vi "Main.vi"() -> ()   [LabVIEW 2020]
doc: "Use this template to build a simple state machine design pattern. Each state executes code and determines which state to transition to."
uses:
  controls/String Selector Control.ctl
  controls/State.ctl
  <vilib>/express/express analysis/Spectral/Block/exnSpectralBlock spectral measurements peak poly.vi
  <vilib>/express/express analysis/Spectral/Block/exnSpectralBlock spectral measurements peak DDT.vi
  <vilib>/express/express analysis/Spectral/XNode/ExpressSpectralMeasurementsBlockNode.xnode
panel:
  in  "Chord Detector":bool
  in  "Single String Tuning":bool
  in  "Mode Switch":bool
  out "Frequency Spectrum":dynamicdata(graph)
  in  "String Selector":T1
  out "Chord":T2
  out "Note":T3
  out "Tuner":T4
  in  "Exit":bool
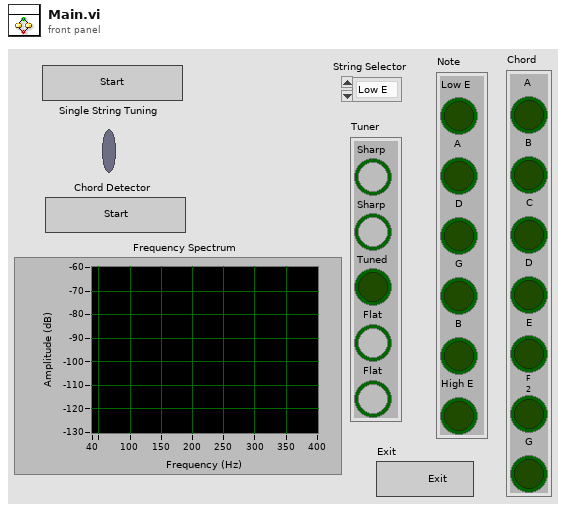
[diagram p1: front panel]
types:
  T1 = typedef "String Selector Control.ctl" = enum16{"Low E", "A", "D", "G", "B", "High E"}
  T2 = cluster{"A":bool, "B":bool, "C":bool, "D":bool, "E":bool, "F 2":bool, "G":bool}
  T3 = cluster{"Low E":bool, "A":bool, "D":bool, "G":bool, "B":bool, "High E":bool}
  T4 = cluster{"Sharp":bool, "Sharp":bool, "Tuned":bool, "Flat":bool, "Flat":bool}
  T5 = cluster{"Tuner":cluster{"Sharp":bool, "Sharp":bool, "Tuned":bool, "Flat":bool, "Flat":bool}, "Chord":cluster{"A":bool, "B":bool, "C":bool, "D":bool, "E":bool, "F 2":bool, "G":bool}, "Note":cluster{"Low E":bool, "A":bool, "D":bool, "G":bool, "B":bool, "High E":bool}, "Frequency Spectrum 2":dynamicdata}
  T6 = typedef "State.ctl" = enum16{"Initialize", "Wait for Event", "Data Acquisition", "Single String", "Chord", "Exit"}
  T7 = cluster{"averaging mode":u16, "weighting mode":u16, "number of averages":u32}
  T8 = cluster{"dB On (F)":bool, "unwrap phase (F)":bool, "convert to degree (F)":bool}
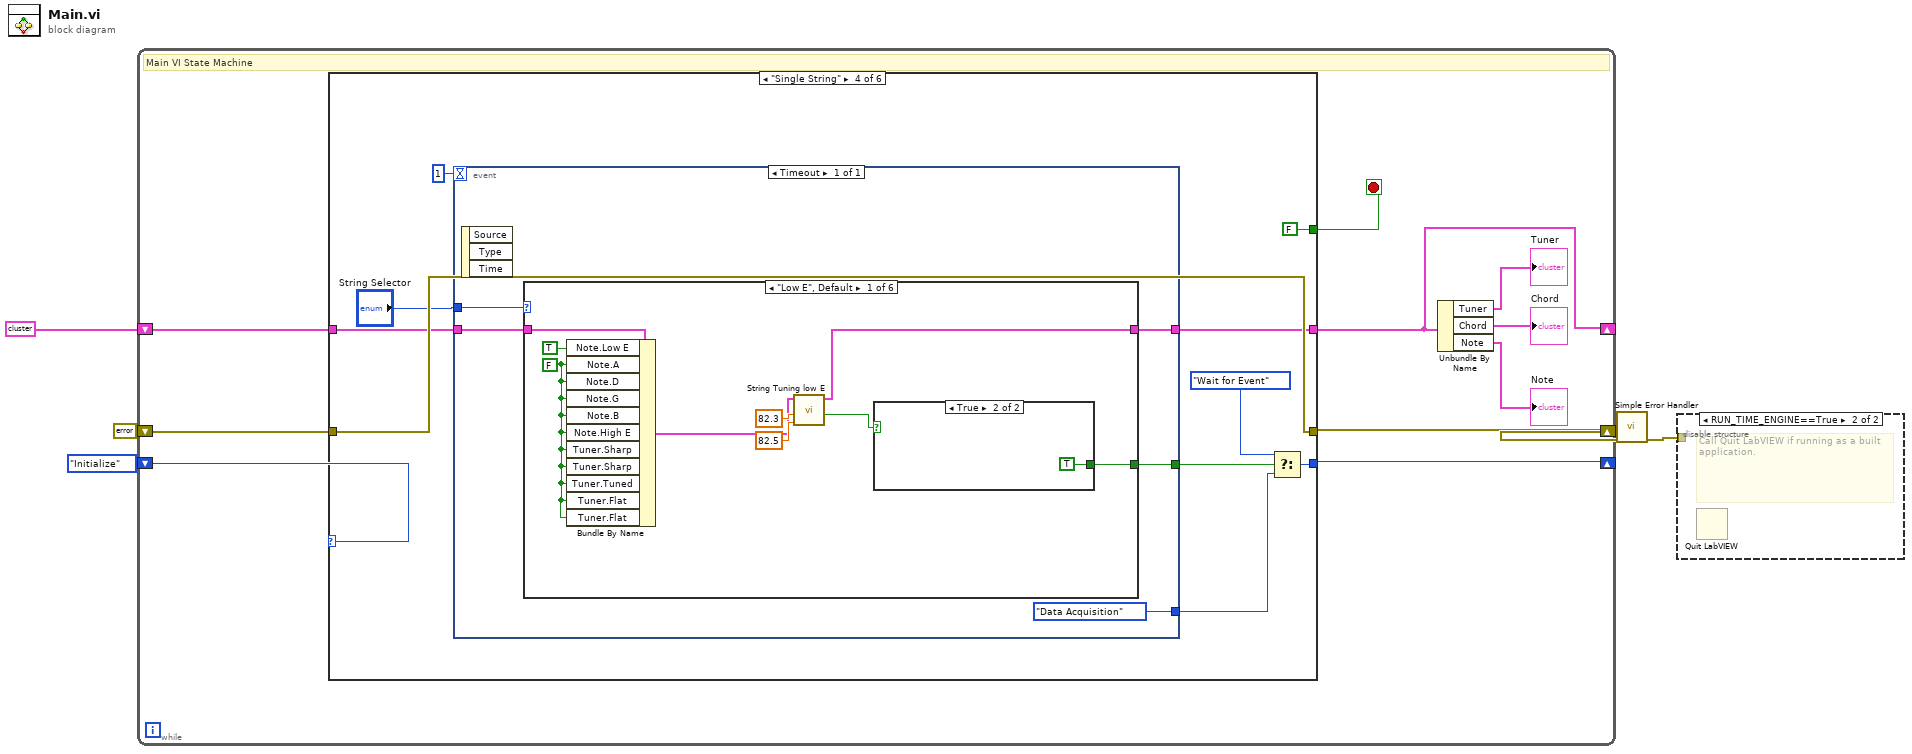
[diagram p0: block diagram]
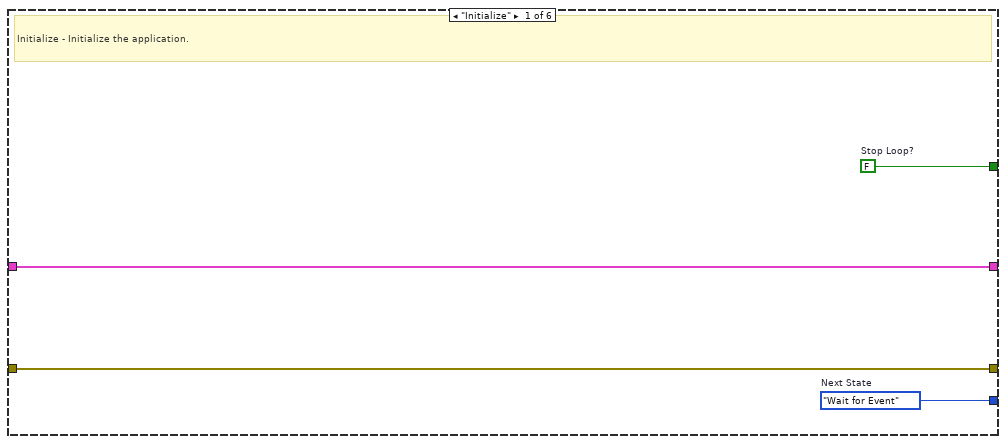
[diagram p3: hidden frame]
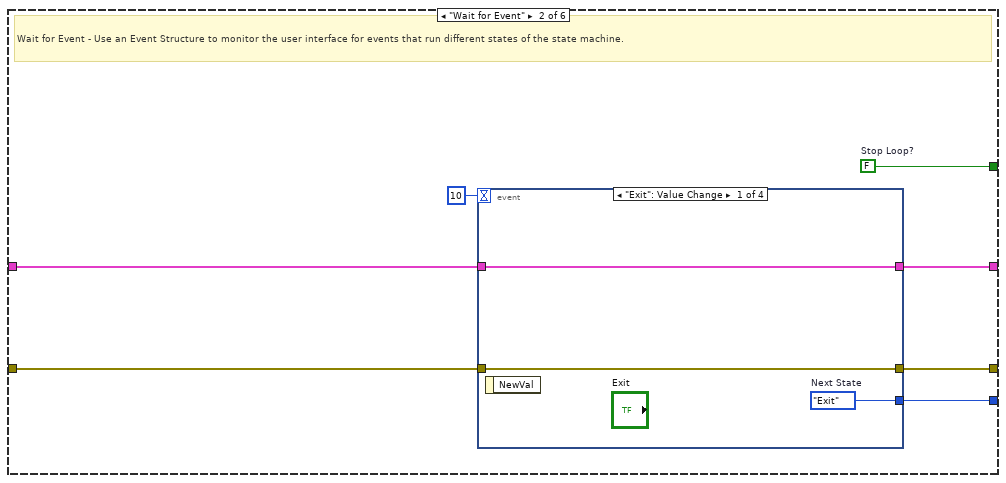
[diagram p4: hidden frame]
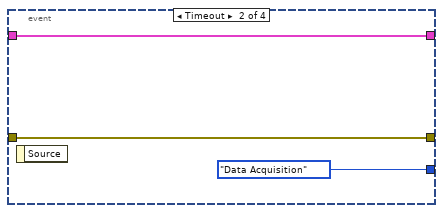
[diagram p5: hidden frame]
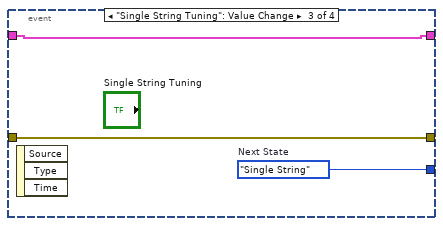
[diagram p6: hidden frame]
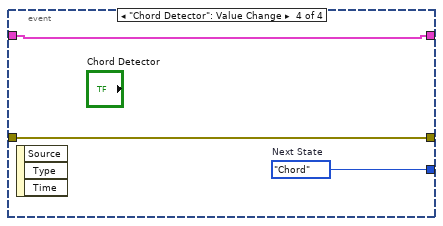
[diagram p7: hidden frame]
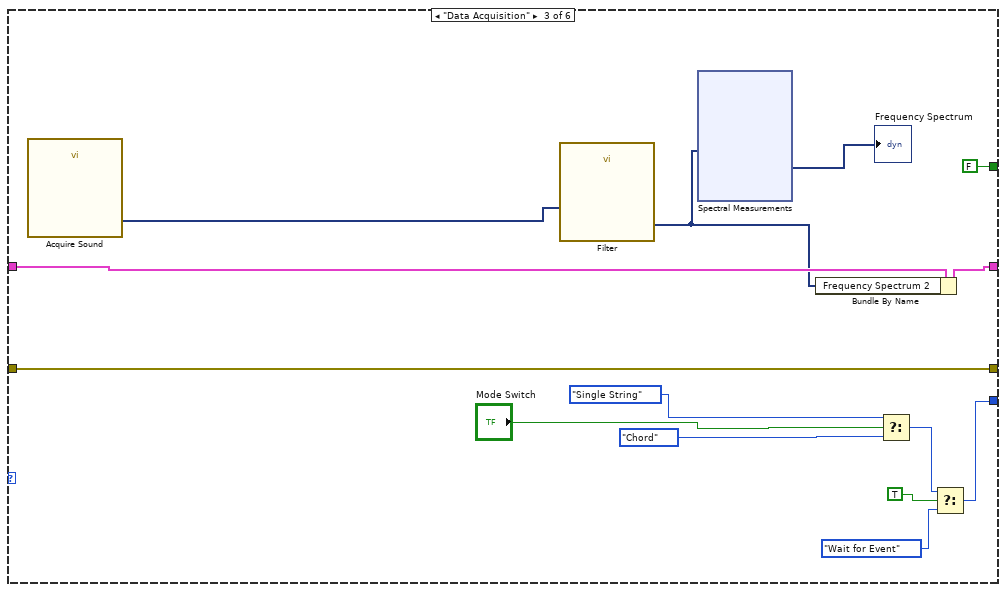
[diagram p8: hidden frame]
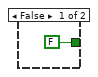
[diagram p9: hidden frame]
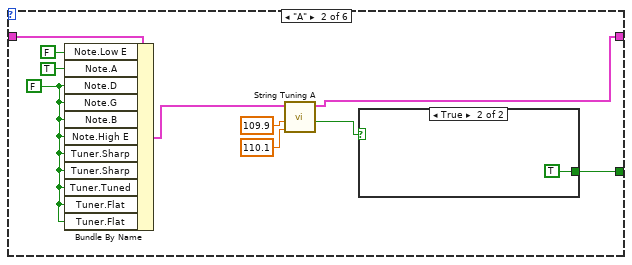
[diagram p10: hidden frame]
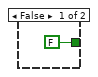
[diagram p11: hidden frame]
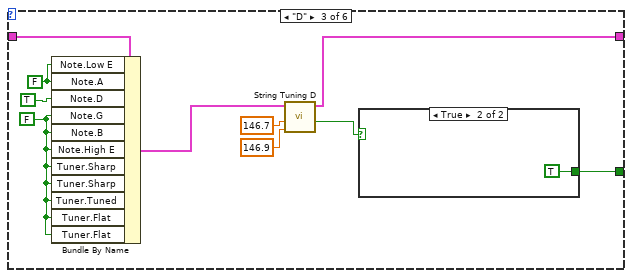
[diagram p12: hidden frame]
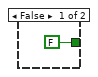
[diagram p13: hidden frame]
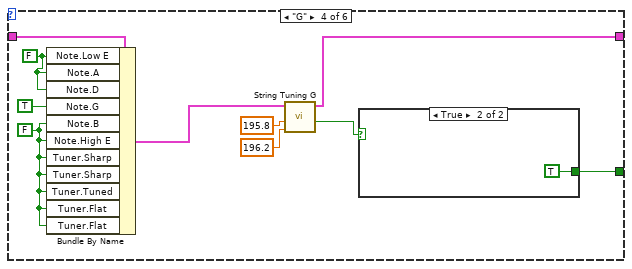
[diagram p14: hidden frame]
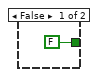
[diagram p15: hidden frame]
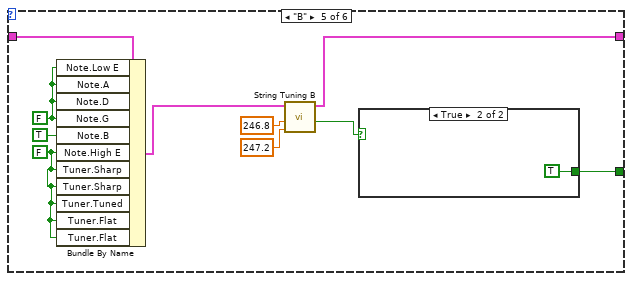
[diagram p16: hidden frame]
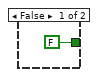
[diagram p17: hidden frame]
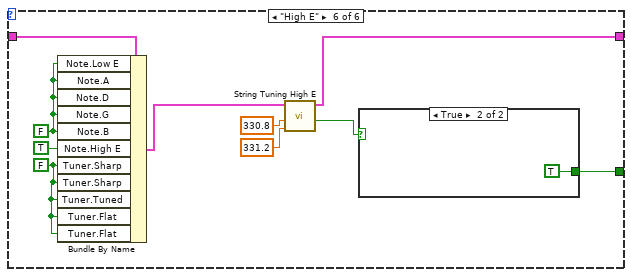
[diagram p18: hidden frame]
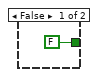
[diagram p19: hidden frame]
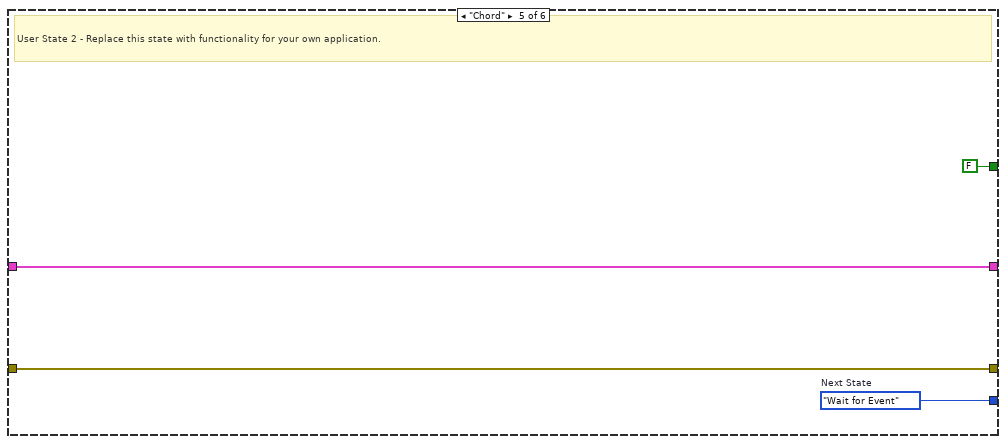
[diagram p20: hidden frame]
diagram:
  n1 = while {
    shift-right: [w14] -> _
    shift-left: State."Initialize" ("Initial State") -> [w15]
    shift-right: [w10] -> _
    shift-left: T5 {"Tuner"={"Sharp"=FALSE, "Sharp"=FALSE, "Tuned"=FALSE, "Flat"=FALSE, "Flat"=FALSE}, "Chord"={"A"=FALSE, "B"=FALSE, "C"=FALSE, "D"=FALSE, "E"=FALSE, "F 2"=FALSE, "G"=FALSE}, "Note"={"Low E"=FALSE, "A"=FALSE, "D"=FALSE, "G"=FALSE, "B"=FALSE, "High E"=FALSE}, "Frequency Spectrum 2"=[{"t0"=timestamp(3721854148.349081 s since 1904-01-01), "dt"=0.0003333, "Y"=array[1000 elements], "attributes"=variant("NI_ChannelName"=variant(string "Voltage"), "NI_UnitDescription"=variant(string "Volts"))}]} ("Input Cluster") -> [w13]
    shift-right: [w11] -> w2
    shift-left: errorcluster {"status"=FALSE, "code"=0, "source"=""} ("error constant") -> [w12]
    stop <- w6 stop-if-true
    # "Main VI State Machine"
    n2 = case shown="\"Single String\"" w15 {
      tunnel: [w19 w26 w48 w69 w152 State."Exit" ("(Value Not Used)")] -> w14
      tunnel: [w18 w25 FALSE ("Stop Loop?") FALSE ("Stop Loop?") FALSE ("Stop Loop?") TRUE ("Stop Loop?")] -> w6
      tunnel: w13 -> [w16 w24 w49 w70 w149 w156]
      tunnel: [w16 w23 w50 w63 w149 w156] -> w10
      tunnel: w12 -> [w17 w22 w52 w72 w150 w155]
      tunnel: [w17 w21 w52 w72 w150 w155] -> w11
      frame "Initialize" {
        w18 = FALSE  # Stop Loop?
        w19 = State."Wait for Event"  # Next State
        # "Initialize - Initialize the application."
      }
      frame "Wait for Event" {
        w25 = FALSE  # Stop Loop?
        # "Wait for Event - Use an Event Structure to monitor the user interface for events that run different states of the state machine."
        n3 = event shown="[0] \"Exit\": Value Change" {
          selector: _ -> [_ _ _ _]
          dyn-events: _ -> [_ _ _ _]
          timeout: 10 -> [_ _ _ _]
          tunnel: [w29 State."Data Acquisition" ("Next State") w35 w38] -> w26
          tunnel: w24 -> [w28 w32 w33 w36]
          tunnel: [w28 w32 w33 w36] -> w23
          tunnel: w22 -> [w27 w31 w34 w37]
          tunnel: [w27 w31 w34 w37] -> w21
          event "Exit": Value Change {
            w29 = State."Exit"  # Next State
            n4 = event-data() -> ()  [unwired: 1 in, 1 out]
          }
          event Timeout {
            n5 = event-data() -> ()  [unwired: 1 in, 1 out]
          }
          event "Single String Tuning": Value Change {
            w35 = State."Single String"  # Next State
            n6 = event-data() -> ()  [unwired: 1 in, 3 out]
          }
          event "Chord Detector": Value Change {
            w38 = State."Chord"  # Next State
            n7 = event-data() -> ()  [unwired: 1 in, 3 out]
          }
        }
      }
      frame "Data Acquisition" {
        n8 = call "Acquire Sound"() -> ("Data"=w40:dynamicdata)  [unwired: 18 in, 1 out]
        n9 = call "Filter"("Signal"=w40) -> ("Filtered Signal"=w42:dynamicdata)  [unwired: 9 in, 1 out]
        n10 = xnode "Spectral Measurements"("Signals"=w42) -> ("FFT - (Peak)"=→"Frequency Spectrum":dynamicdata)  [unwired: 1 in, 2 out]
        n11 = Bundle By Name(cluster=w49, "Frequency Spectrum 2"=w42) -> (w50:T5)
        n12 = Select(t=State."Single String" ("(Value Not Used)"), s="Mode Switch", f=State."Chord" ("(Value Not Used)")) -> (s? t:f=w44:T6)
        n13 = Select(t=w44, s=TRUE, f=State."Wait for Event" ("(Value Not Used)")) -> (s? t:f=w48:T6)
      }
      frame "Single String" {
        n14 = event shown="[0] Timeout" {
          selector: _ -> [_]
          dyn-events: _ -> [_]
          timeout: 1 -> [_]
          tunnel: "String Selector" -> [w77]
          tunnel: [w76] -> w63
          tunnel: w70 -> [w75]
          tunnel: [w74] -> w65
          tunnel: [State."Data Acquisition" ("f")] -> w64
          event Timeout {
            n15 = event-data() -> ()  [unwired: 1 in, 3 out]
            n16 = case shown="\"Low E\", Default" w77 {
              tunnel: [w84 w89 w101 w113 w125 w137] -> w76
              tunnel: w75 -> [w79 w92 w106 w118 w130 w142]
              tunnel: [w82 w95 w107 w120 w132 w144] -> w74
              frame "Low E", Default {
                w78 = FALSE ("Note.A")
                n17 = Bundle By Name(cluster=w79, "Note.Low E"=TRUE, "Note.A"=w78, "Note.D"=w78, "Note.G"=w78, "Note.B"=w78, "Note.High E"=w78, "Tuner.Sharp"=w78, "Tuner.Sharp"=w78, "Tuner.Tuned"=w78, "Tuner.Flat"=w78, "Tuner.Flat"=w78) -> (w80:T5)
                n18 = call "String Tuning low E.vi"("Upper Limit"=82.5 ("y"), "Lower Limit"=82.3 ("y"), "Input Cluster"=w80) -> ("Tuned"=w83:bool, "Output Cluster"=w84:T5)  [unwired: 7 in]
                n19 = case shown="True" w83 {
                  tunnel: [FALSE TRUE] -> w82
                  frame False {
                  }
                  frame True {
                  }
                }
              }
              frame "A" {
                w91 = FALSE ("Note.D")
                n20 = Bundle By Name(cluster=w92, "Note.Low E"=FALSE, "Note.A"=TRUE, "Note.D"=w91, "Note.G"=w91, "Note.B"=w91, "Note.High E"=w91, "Tuner.Sharp"=w91, "Tuner.Sharp"=w91, "Tuner.Tuned"=w91, "Tuner.Flat"=w91, "Tuner.Flat"=w91) -> (w90:T5)
                n21 = call "String Tuning A.vi"("Upper Limit"=110.1 ("y"), "Lower Limit"=109.9 ("y"), "Input Cluster"=w90) -> ("Tuned"=w96:bool, "Output Cluster"=w89:T5)  [unwired: 7 in]
                n22 = case shown="True" w96 {
                  tunnel: [FALSE TRUE] -> w95
                  frame False {
                  }
                  frame True {
                  }
                }
              }
              frame "D" {
                w103 = FALSE ("Note.Low E")
                w104 = FALSE ("Note.A")
                n23 = Bundle By Name(cluster=w106, "Note.Low E"=w104, "Note.A"=w104, "Note.D"=TRUE ("Note.A"), "Note.G"=w103, "Note.B"=w103, "Note.High E"=w103, "Tuner.Sharp"=w103, "Tuner.Sharp"=w103, "Tuner.Tuned"=w103, "Tuner.Flat"=w103, "Tuner.Flat"=w103) -> (w102:T5)
                n24 = call "String Tuning D.vi"("Upper Limit"=146.9 ("y"), "Lower Limit"=146.7 ("y"), "Input Cluster"=w102) -> ("Tuned"=w108:bool, "Output Cluster"=w101:T5)  [unwired: 7 in]
                n25 = case shown="True" w108 {
                  tunnel: [FALSE TRUE] -> w107
                  frame False {
                  }
                  frame True {
                  }
                }
              }
              frame "G" {
                w115 = FALSE
                w117 = FALSE ("Note.Low E")
                n26 = Bundle By Name(cluster=w118, "Note.Low E"=w117, "Note.A"=w117, "Note.D"=w117, "Note.G"=TRUE, "Note.B"=w115, "Note.High E"=w115, "Tuner.Sharp"=w115, "Tuner.Sharp"=w115, "Tuner.Tuned"=w115, "Tuner.Flat"=w115, "Tuner.Flat"=w115) -> (w114:T5)
                n27 = call "String Tuning G.vi"("Upper Limit"=196.2 ("y"), "Lower Limit"=195.8 ("y"), "Input Cluster"=w114) -> ("Tuned"=w119:bool, "Output Cluster"=w113:T5)  [unwired: 7 in]
                n28 = case shown="True" w119 {
                  tunnel: [FALSE TRUE] -> w120
                  frame False {
                  }
                  frame True {
                  }
                }
              }
              frame "B" {
                w127 = FALSE ("Note.G")
                w128 = FALSE ("Note.High E")
                n29 = Bundle By Name(cluster=w130, "Note.Low E"=w127, "Note.A"=w127, "Note.D"=w127, "Note.G"=w127, "Note.B"=TRUE, "Note.High E"=w128, "Tuner.Sharp"=w128, "Tuner.Sharp"=w128, "Tuner.Tuned"=w128, "Tuner.Flat"=w128, "Tuner.Flat"=w128) -> (w126:T5)
                n30 = call "String Tuning B.vi"("Upper Limit"=247.2 ("y"), "Lower Limit"=246.8 ("y"), "Input Cluster"=w126) -> ("Tuned"=w131:bool, "Output Cluster"=w125:T5)  [unwired: 7 in]
                n31 = case shown="True" w131 {
                  tunnel: [FALSE TRUE] -> w132
                  frame False {
                  }
                  frame True {
                  }
                }
              }
              frame "High E" {
                w139 = FALSE ("Note.B")
                w140 = FALSE ("Tuner.Sharp")
                n32 = Bundle By Name(cluster=w142, "Note.Low E"=w139, "Note.A"=w139, "Note.D"=w139, "Note.G"=w139, "Note.B"=w139, "Note.High E"=TRUE, "Tuner.Sharp"=w140, "Tuner.Sharp"=w140, "Tuner.Tuned"=w140, "Tuner.Flat"=w140, "Tuner.Flat"=w140) -> (w138:T5)
                n33 = call "String Tuning High E.vi"("Upper Limit"=331.2 ("y"), "Lower Limit"=330.8 ("y"), "Input Cluster"=w138) -> ("Tuned"=w143:bool, "Output Cluster"=w137:T5)  [unwired: 7 in]
                n34 = case shown="True" w143 {
                  tunnel: [FALSE TRUE] -> w144
                  frame False {
                  }
                  frame True {
                  }
                }
              }
            }
          }
        }
        n35 = Select(t=State."Wait for Event" ("(Value Not Used)"), s=w65, f=w64) -> (s? t:f=w69:T6)
      }
      frame "Chord" {
        w152 = State."Wait for Event"  # Next State
        # "User State 2 - Replace this state with functionality for your own application."
      }
      frame "Exit" {
      }
    }
    n36 = Unbundle By Name(w10) -> ("Tuner"=→"Tuner":T4, "Chord"=→"Chord":T2, "Note"=→"Note":T3)
  }
  n37 = call <vilib>:"Simple Error Handler.vi"("error in (no error)"=w2) -> ("error out"=w4:errorcluster)  [unwired: 4 in, 4 out]
  n38 = disable-structure shown="RUN_TIME_ENGINE==True" {
    disable-tunnel: w4 -> [_ _]
    frame condition #0 (active) {
    }
    frame condition #1 {
      # "Call Quit LabVIEW if running as a built application."
      n39 = Quit LabVIEW() -> ()  [unwired: 1 in]
    }
  }
